vi "Morse_Decoder.vi"() -> ()   [LabVIEW 2024]
uses:
  <vilib>/DAQmx/read.llb/DAQmx Read (Analog 2D DBL NChan NSamp).vi
  <vilib>/DAQmx/create/channels.llb/DAQmx Create Channel (AI-Voltage-Basic).vi
  <vilib>/DAQmx/configure/timing.llb/DAQmx Timing (Sample Clock).vi
  <vilib>/DAQmx/miscellaneous.llb/DAQmx Fill In Error Info.vi
panel:
  out "output variable":i32[](array[numeric])
  out "String Pre Procesare":string
  out "result_out":i32[](array[numeric])
  out "size(s)":i32
  out "result_len":i32
  out "morse_len":dbl
  in  "Tab Control":enum32{"TAB"}(tab)
  out "Decoded message":i16[](graph)
  out "Trigger view":waveform(dbl)(graph)={"t0"=timestamp(0 s since 1904-01-01), "dt"=0.0002, "Y"=[]}
  out "TX":bool
  in  "StartRX":bool=TRUE
  in  "ClearMsgBuffer":bool
  in  "STOP":bool
  in  "sample mode":i32(ring)=10178 items=["Finite Samples"=10178, "Continuous Samples"=10123, "Hardware Timed Single Point"=12522]
  in  "physical channels":tag="Dev2/ai0"
  in  "input terminal configuration":i32(ring)=10083 items=["default"=-1, "RSE"=10083, "NRSE"=10078, "Differential"=10106, "Pseudodifferential"=12529]
  in  "maximum value":dbl=5.0 format="%0.2f"
  in  "minimum value":dbl=-5.0 format="%0.2f"
  in  "milliseconds to wait":u32=10
  in  "Prag":dbl(knob)=0.1 scale=0.0..5.0
  in  "samples per channel":i32=50
  in  "rate":dbl=5000.0 format="%0.2f"
  in  "timeout":dbl=10.0 format="%0.2f"
  in  "number of samples per channel":i32=50
  out "perioada":dbl
  out "error out":errorcluster
  out "MESSAGE ARRAY SIZE":i32
  out "READ BUFFER SIZE":i32=302
  out "TXStopBuff":dbl=24.0
  out "INTERMIDIATE BUFFER":dbl[](array[numeric])
  out "READ BUFFER":dbl[](array[numeric])
  out "MESSAGE ARRAY":bool[](array[boolean])
  out "Message points":bool[](array[boolean])
  out "dbg lamp":bool
  out "TrueCnt":i32
  in  "Clear String":bool
  out "Message":string
  # "INPUT CONFIG"
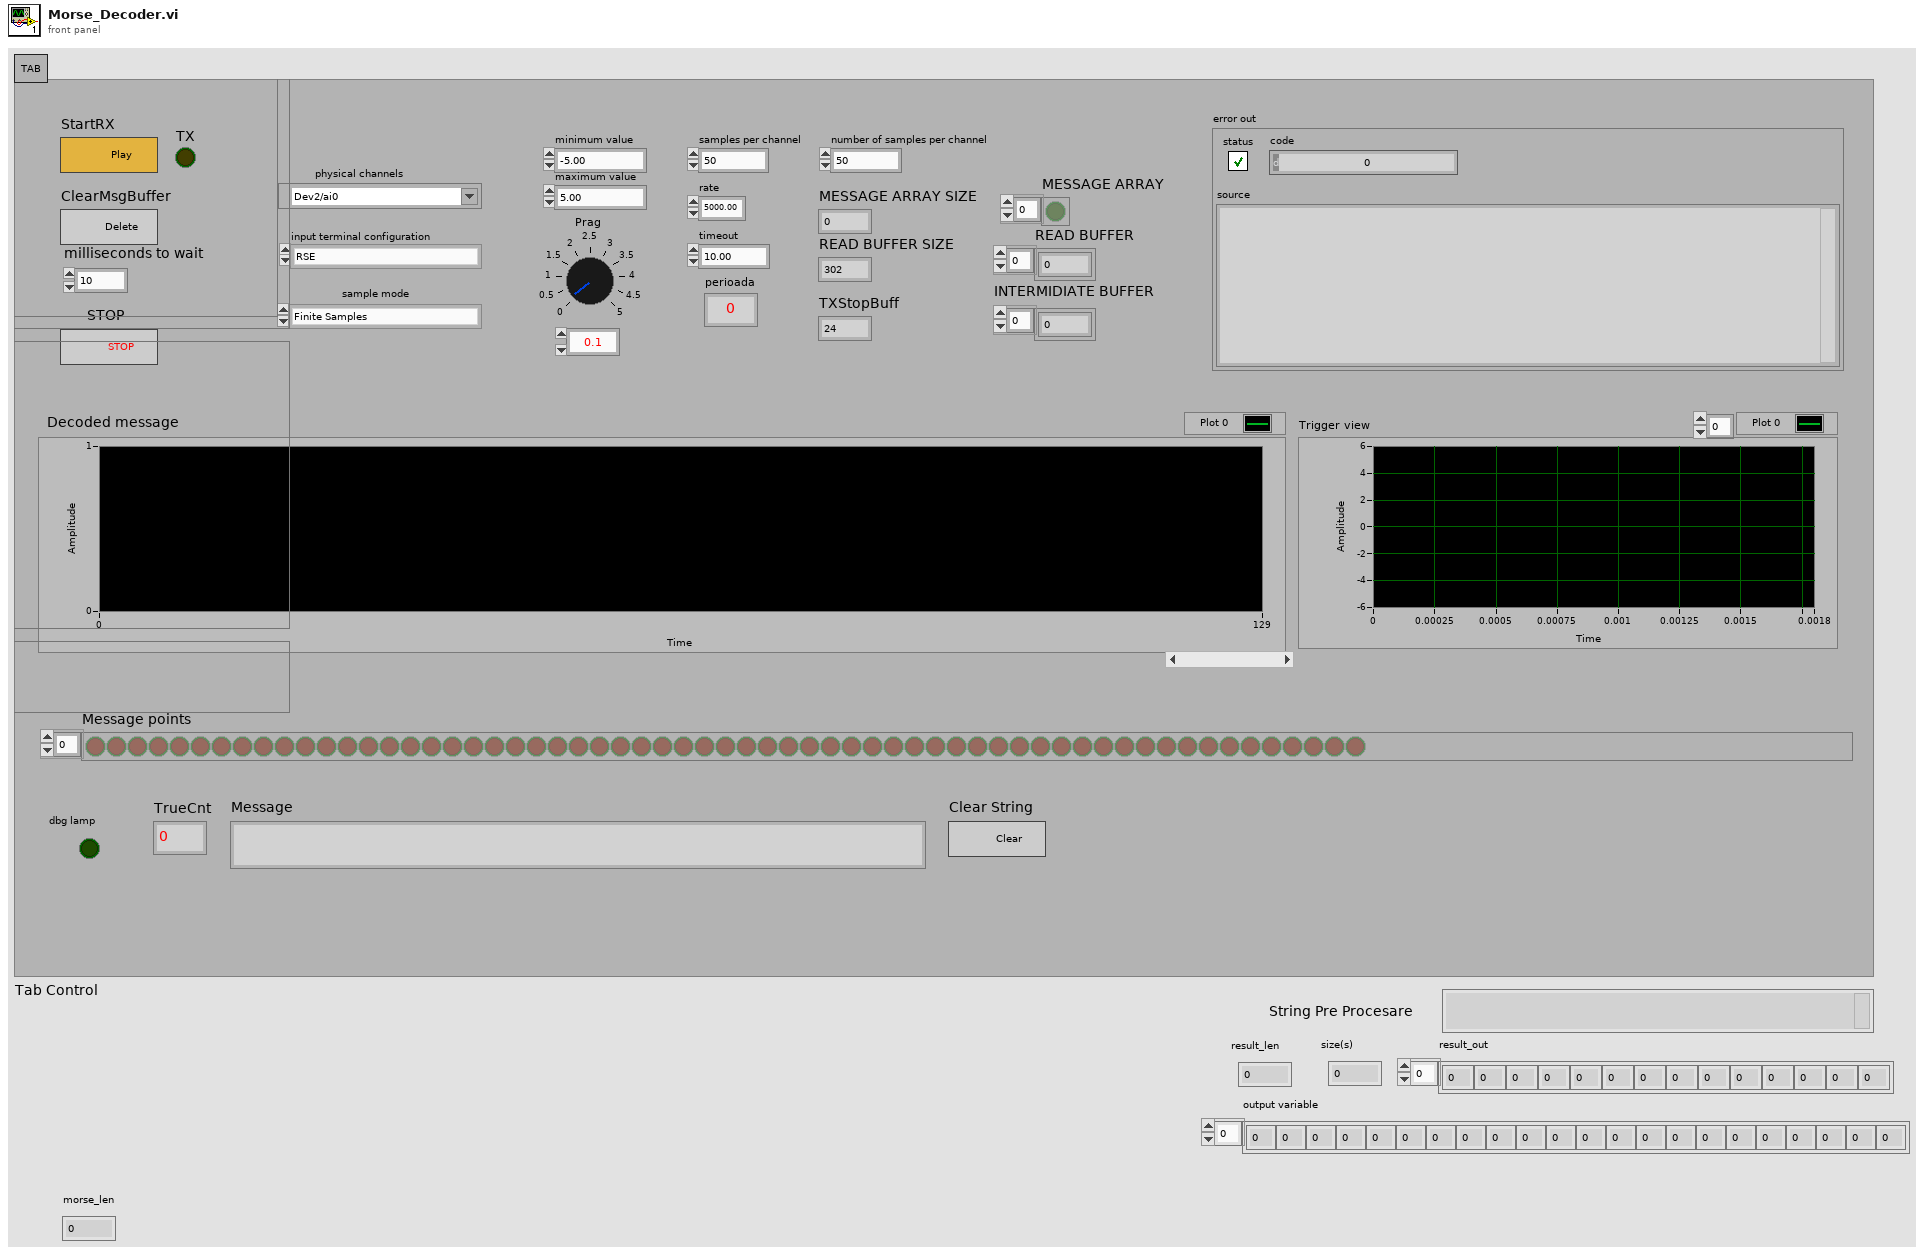
[diagram p1: front panel]
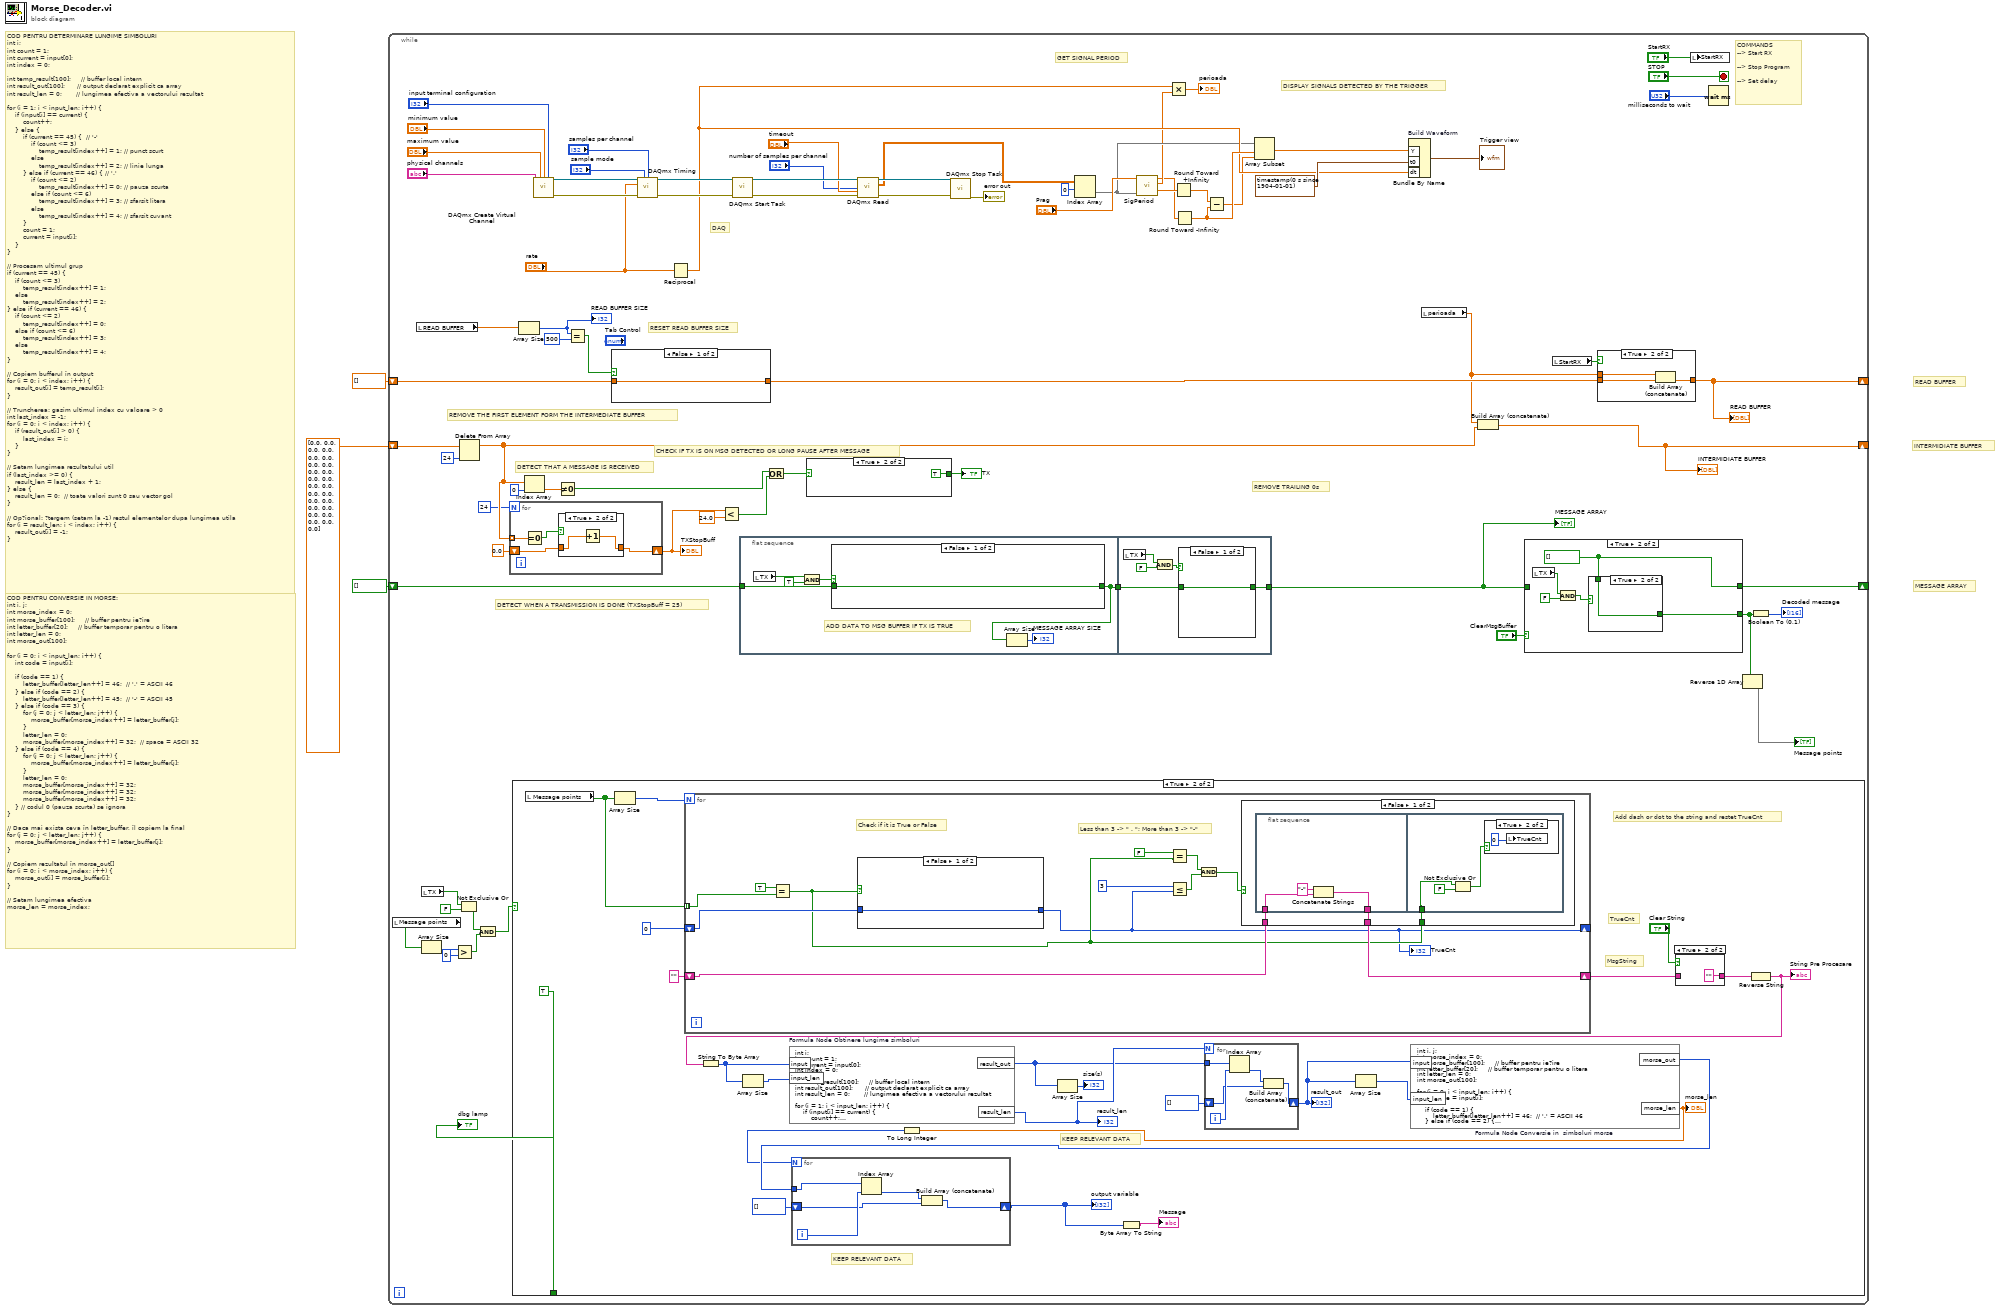
[diagram p0: block diagram]
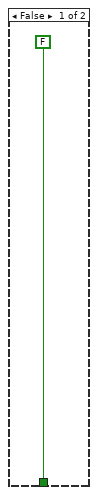
[diagram p2: hidden frame]
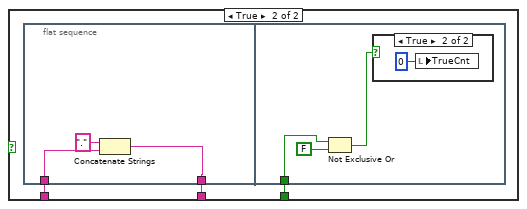
[diagram p5: hidden frame]
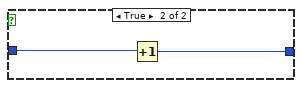
[diagram p7: hidden frame]
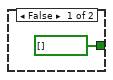
[diagram p9: hidden frame]
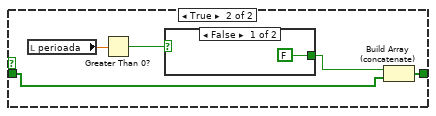
[diagram p10: hidden frame]
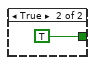
[diagram p11: hidden frame]
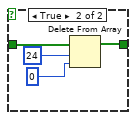
[diagram p12: hidden frame]
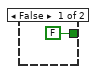
[diagram p15: hidden frame]
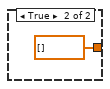
[diagram p16: hidden frame]
diagram:
  # "COD PENTRU CONVERSIE IN MORSE:\nint i, j;\nint morse_index = 0;\nint morse_buffer[100];     // buffer pentru ie?ire\nint letter_buffer[20];     // buffer temporar pentru o litera\nint letter_len = 0;\nint morse_out[100];\n\nfor (i = 0; i < input_len; i++) {\n    int code = input[i];\n\n    if (code == 1) {\n        letter_buffer[letter_len++] = 46;  // '.' = ASCII 46\n    } else if (code == 2) {\n        letter_buffer[letter_len++] = 45;  // '-' = ASCII 45\n    } else if (code == 3) {\n        for (j = 0; j < letter_len; j++) {\n            morse_buffer[morse_index++] = letter_buffer[j];\n        }\n        letter_len = 0;\n        morse_buffer[morse_index++] = 32;  // space = ASCII 32\n    } else if (code == 4) {\n        for (j = 0; j < letter_len; j++) {\n            morse_buffer[morse_index++] = letter_buffer[j];\n        }\n        letter_len = 0;\n        morse_buffer[morse_index++] = 32;\n        morse_buffer[morse_index++] = 32;\n        morse_buffer[morse_index++] = 32;\n    } // codul 0 (pauza scurta) se ignora\n}\n\n// Daca mai exista ceva în letter_buffer, îl copiem la final\nfor (j = 0; j < letter_len; j++) {\n    morse_buffer[morse_index++] = letter_buffer[j];\n}\n\n// Copiem rezultatul în morse_out[]\nfor (i = 0; i < morse_index; i++) {\n    morse_out[i] = morse_buffer[i];\n}\n\n// Setam lungimea efectiva\nmorse_len = morse_index;"
  # "COD PENTRU DETERMINARE LUNGIME SIMBOLURI\nint i;\nint count = 1;\nint current = input[0];\nint index = 0;\n\nint temp_result[100];     // buffer local intern\nint result_out[100];      // output declarat explicit ca array\nint result_len = 0;       // lungimea efectiva a vectorului rezultat\n\nfor (i = 1; i < input_len; i++) {\n    if (input[i] == current) {\n        count++;\n    } else {\n        if (current == 45) {  // '-'\n            if (count <= 3)\n                temp_result[index++] = 1; // punct scurt\n            else\n                temp_result[index++] = 2; // linie lunga\n        } else if (current == 46) { // '.'\n            if (count <= 2)\n                temp_result[index++] = 0; // pauza scurta\n            else if (count <= 6)\n                temp_result[index++] = 3; // sfarsit litera\n            else\n                temp_result[index++] = 4; // sfarsit cuvant\n        }\n        count = 1;\n        current = input[i];\n    }\n}\n\n// Procesam ultimul grup\nif (current == 45) {\n    if (count <= 3)\n        temp_result[index++] = 1;\n    else\n        temp_result[index++] = 2;\n} else if (current == 46) {\n    if (count <= 2)\n        temp_result[index++] = 0;\n    else if (count <= 6)\n        temp_result[index++] = 3;\n    else\n        temp_result[index++] = 4;\n}\n\n// Copiem bufferul în output\nfor (i = 0; i < index; i++) {\n    result_out[i] = temp_result[i];\n}\n\n// Truncherea: gasim ultimul index cu valoare > 0\nint last_index = -1;\nfor (i = 0; i < index; i++) {\n    if (result_out[i] > 0) {\n        last_index = i;\n    }\n}\n\n// Setam lungimea rezultatului util\nif (last_index >= 0) {\n    result_len = last_index + 1;\n} else {\n    result_len = 0;  // toate valori sunt 0 sau vector gol\n}\n\n// Op?ional: ?tergem (setam la -1) restul elementelor dupa lungimea utila\nfor (i = result_len; i < index; i++) {\n    result_out[i] = -1;\n}"
  # "INTERMIDIATE BUFFER"
  # "READ BUFFER"
  # "MESSAGE ARRAY"
  n1 = while {
    shift-right: [w17] -> _
    shift-left: bool[] [] -> [w20]
    shift-right: [w44] -> _
    shift-left: dbl[] [] -> [w41]
    shift-right: [w35] -> _
    shift-left: dbl[] [0.0, 0.0, 0.0, 0.0, 0.0, 0.0, 0.0, 0.0, 0.0, 0.0, 0.0, 0.0, 0.0, 0.0, 0.0, 0.0, 0.0, 0.0, 0.0, 0.0, 0.0, 0.0, 0.0, 0.0, 0.0] -> [w36]
    stop <- "STOP" stop-if-true
    # "REMOVE TRAILING 0s"
    # "COMMANDS\n--> Start RX\n\n--> Stop Program\n\n--> Set delay"
    # "REMOVE THE FIRST ELEMENT FORM THE INTERMEDIATE BUFFER"
    # "DAQ"
    # "GET SIGNAL PERIOD"
    # "DISPLAY SIGNALS DETECTED BY THE TRIGGER"
    # "CHECK IF TX IS ON MSG DETECTED OR LONG PAUSE AFTER MESSAGE"
    # "DETECT WHEN A TRANSMISSION IS DONE (TXStopBuff = 25)"
    # "DETECT THAT A MESSAGE IS RECEIVED"
    # "RESET READ BUFFER SIZE"
    n2 = local read "Message points"() -> (w10:bool[])
    n3 = local read "READ BUFFER"() -> (w39:dbl[])
    n4 = local read "TX"() -> (w11:bool)
    n5 = Array Size(array=w10) -> (size(s)=w9:i32)
    n6 = Greater?(x=w9, y=0) -> (0:w6:bool)
    n7 = Not Exclusive Or(1:FALSE ("y"), 2:w11) -> (0:w7:bool)
    n8 = Delete From Array(array=w36, index=24) -> (array with subset deleted=w30:dbl[])  [unwired: 1 in, 1 out]
    n9 = And(x=w7, y=w6) -> (x .and. y?=w5:bool)
    n10 = for {
      N: 24 -> [_]
      shift-right: [w187] -> w25
      shift-left: 0.0 -> [w188]
      tunnel: w30 -> [w190] mode=indexing
      n11 = Equal To 0?(x=w190) -> (x = 0?=w189:bool)
      n12 = case shown="True" w189 {
        tunnel: w188 -> [w191 w193]
        tunnel: [w191 w192] -> w187
        frame False {
        }
        frame True {
          n13 = Increment(x=w193) -> (x+1=w192:dbl)
        }
      }
    }
    "TXStopBuff" <- w25
    n14 = case shown="True" w5 {
      tunnel: [FALSE TRUE] -> w4
      frame False {
      }
      frame True {
        # "KEEP RELEVANT DATA"
        # "KEEP RELEVANT DATA"
        # "Add dash or dot to the string and restet TrueCnt"
        # "MsgString"
        # "TrueCnt"
        n15 = local read "Message points"() -> (w101:bool[])
        n16 = Array Size(array=w101) -> (size(s)=w103:i32)
        n17 = for {
          N: w103 -> [_]
          shift-right: [w122] -> w100
          shift-left: "" -> [w123]
          shift-right: [w116] -> _
          shift-left: 0 -> [w125]
          tunnel: w101 -> [w127] mode=indexing
          # "Less than 3 -> \" . \"; More than 3 -> \"-\""
          # "Check if it is True or False"
          n18 = Equal?(x=TRUE, y=w127) -> (x = y?=w121:bool)
          n19 = case shown="False" w121 {
            tunnel: w125 -> [w148 w150]
            tunnel: [w148 w149] -> w116
            frame False {
            }
            frame True {
              n20 = Increment(x=w150) -> (x+1=w149:i32)
            }
          }
          "TrueCnt" <- w116
          n21 = Equal?(x=FALSE, y=w121) -> (x = y?=w119:bool)
          n22 = Less Or Equal?(x=3, y=w116) -> (x <= y?=w118:bool)
          n23 = And(x=w119, y=w118) -> (x .and. y?=w117:bool)
          n24 = case shown="False" w117 {
            tunnel: w123 -> [w130 w140]
            tunnel: [w129 w139] -> w122
            tunnel: w121 -> [w128 w138]
            frame False {
              n25 = flat-sequence {
                tunnel: w130 -> [w133]
                tunnel: [w132] -> w129
                tunnel: w128 -> [w134]
                frame #0 {
                  n26 = Concatenate Strings("-" ("string"), w133) -> (w132:string)
                }
                frame #1 {
                  n27 = Not Exclusive Or(1:FALSE ("y"), 2:w134) -> (0:w136:bool)
                  n28 = case shown="True" w136 {
                    frame False {
                    }
                    frame True {
                      n29 = local write "TrueCnt"(0) -> ()
                    }
                  }
                }
              }
            }
            frame True {
              n30 = flat-sequence {
                tunnel: [w142] -> w139
                tunnel: w140 -> [w143]
                tunnel: w138 -> [w144]
                frame #0 {
                  n31 = Concatenate Strings("." ("string"), w143) -> (w142:string)
                }
                frame #1 {
                  n32 = Not Exclusive Or(1:FALSE ("y"), 2:w144) -> (0:w146:bool)
                  n33 = case shown="True" w146 {
                    frame False {
                    }
                    frame True {
                      n34 = local write "TrueCnt"(0 ("TrueCnt")) -> ()
                    }
                  }
                }
              }
            }
          }
        }
        n35 = case shown="True" "Clear String" {
          tunnel: w100 -> [w114 _]
          tunnel: [w114 ""] -> w97
          frame False {
          }
          frame True {
          }
        }
        n36 = Reverse String(1:w97) -> (0:w93:string)
        "String Pre Procesare" <- w93
        n37 = String To Byte Array(string=w93) -> (unsigned byte array=w95:u8[])
        n38 = Array Size(array=w95) -> (size(s)=w94:i32)
        n39 = formula code="int i;\nint count = 1;\nint current = input[0];\nint index = 0;\n\nint temp_result[100];     // buffer local intern\nint result_out[100];      // output declarat explicit ca array\nint result_len = 0;       // lungimea efectiva a vectorului rezultat\n\nfor (i = 1; i < input_len; i++) {\n    if (input[i] == current) {\n        count++;\n    } else {\n        if (current == 45) {  // '-'\n            if (count <= 3)\n                temp_result[index++] = 1; // punct scurt\n            else\n                temp_result[index++] = 2; // linie lunga\n        } else if (current == 46) { // '.'\n            if (count <= 2)\n                temp_result[index++] = 0; // pauza scurta\n            else if (count <= 6)\n                temp_result[index++] = 3; // sfarsit litera\n            else\n                temp_result[index++] = 4; // sfarsit cuvant\n        }\n        count = 1;\n        current = input[i];\n    }\n}\n\n// Procesam ultimul grup\nif (current == 45) {\n    if (count <= 3)\n        temp_result[index++] = 1;\n    else\n        temp_result[index++] = 2;\n} else if (current == 46) {\n    if (count <= 2)\n        temp_result[index++] = 0;\n    else if (count <= 6)\n        temp_result[index++] = 3;\n    else\n        temp_result[index++] = 4;\n}\n\n// Copiem bufferul în output\nfor (i = 0; i < index; i++) {\n    result_out[i] = temp_result[i];\n}\n\n// Truncherea: gasim ultimul index cu valoare > 0\nint last_index = -1;\nfor (i = 0; i < index; i++) {\n    if (result_out[i] > 0) {\n        last_index = i;\n    }\n}\n\n// Setam lungimea rezultatului util\nif (last_index >= 0) {\n    result_len = last_index + 1;\n} else {\n    result_len = 0;  // toate valori sunt 0 sau vector gol\n}\n\n// Op?ional: ?tergem (setam la -1) restul elementelor dupa lungimea utila\nfor (i = result_len; i < index; i++) {\n    result_out[i] = -1;\n}" "Formula Node Obtinere lungime simboluri"("input"=w95, "input_len"=w94) -> ("result_out"=w90:i32[], "result_len"=w91:i32)
        "result_len" <- w91
        n40 = Array Size(array=w90) -> (size(s)=→"size(s)":i32)
        n41 = for {
          N: w91 -> [_]
          tunnel: w90 -> [w112]
          shift-right: [w109] -> w88
          shift-left: i32[] [] -> [w110]
          i -> [w113]
          n42 = Index Array(array=w112, index=w113) -> (element=w111:i32)
          n43 = Build Array (concatenate)(w111, w110) -> (w109:i32[])
        }
        "result_out" <- w88
        n44 = Array Size(array=w88) -> (size(s)=w87:i32)
        n45 = formula code="int i, j;\nint morse_index = 0;\nint morse_buffer[100];     // buffer pentru ie?ire\nint letter_buffer[20];     // buffer temporar pentru o litera\nint letter_len = 0;\nint morse_out[100];\n\nfor (i = 0; i < input_len; i++) {\n    int code = input[i];\n\n    if (code == 1) {\n        letter_buffer[letter_len++] = 46;  // '.' = ASCII 46\n    } else if (code == 2) {\n        letter_buffer[letter_len++] = 45;  // '-' = ASCII 45\n    } else if (code == 3) {\n        for (j = 0; j < letter_len; j++) {\n            morse_buffer[morse_index++] = letter_buffer[j];\n        }\n        letter_len = 0;\n        morse_buffer[morse_index++] = 32;  // space = ASCII 32\n    } else if (code == 4) {\n        for (j = 0; j < letter_len; j++) {\n            morse_buffer[morse_index++] = letter_buffer[j];\n        }\n        letter_len = 0;\n        morse_buffer[morse_index++] = 32;\n        morse_buffer[morse_index++] = 32;\n        morse_buffer[morse_index++] = 32;\n    } // codul 0 (pauza scurta) se ignora\n}\n\n// Daca mai exista ceva în letter_buffer, îl copiem la final\nfor (j = 0; j < letter_len; j++) {\n    morse_buffer[morse_index++] = letter_buffer[j];\n}\n\n// Copiem rezultatul în morse_out[]\nfor (i = 0; i < morse_index; i++) {\n    morse_out[i] = morse_buffer[i];\n}\n\n// Setam lungimea efectiva\nmorse_len = morse_index;" "Formula Node Conversie in  simboluri morse"("input"=w88, "input_len"=w87) -> ("morse_out"=w85:i32[], "morse_len"=w84:dbl)
        "morse_len" <- w84
        n46 = To Long Integer(number=w84) -> (32bit integer=w83:i32)
        n47 = for {
          N: w83 -> [_]
          shift-right: [w106] -> w81
          shift-left: i32[] [] -> [w104]
          tunnel: w85 -> [w108]
          i -> [w107]
          n48 = Index Array(array=w108, index=w107) -> (element=w105:i32)
          n49 = Build Array (concatenate)(w105, w104) -> (w106:i32[])
        }
        "output variable" <- w81
        n50 = Byte Array To String(unsigned byte array=w81) -> (string=→"Message":string)
      }
    }
    "dbg lamp" <- w4
    n51 = Array Size(array=w39) -> (size(s)=w38:i32)
    "READ BUFFER SIZE" <- w38
    n52 = Index Array(array=w30, index=0) -> (element=w33:dbl)
    n53 = call-poly <vilib>:"DAQmx Create Virtual Channel.vi"("maximum value"="maximum value", "minimum value"="minimum value", "input terminal configuration"="input terminal configuration", "physical channels"="physical channels") -> ("task out"=w74:refnum<k21>, "error out"=w79:errorcluster)  [unwired: 10 in]
    n54 = Not Equal To 0?(x=w33) -> (x != 0?=w26:bool)
    n55 = Equal?(x=w38, y=500) -> (x = y?=w42:bool)
    n56 = case shown="False" w42 {
      tunnel: w41 -> [w196 _]
      tunnel: [w196 dbl[] []] -> w40
      frame False {
      }
      frame True {
      }
    }
    n57 = call-poly <vilib>:"DAQmx Timing.vi"("task/channels in"=w74, "sample mode"="sample mode", "samples per channel"="samples per channel", "rate"="rate", "error in"=w79) -> ("task out"=w73:refnum<k21>, "error out"=w78:errorcluster)  [unwired: 9 in]
    n58 = Reciprocal(x="rate") -> (1/x=w54:dbl)
    n59 = Less?(x=w25, y=24.0) -> (x < y?=w23:bool)
    n60 = call <vilib>:"DAQmx Start Task.vi"("task/channels in"=w73, "error in"=w78) -> ("task out"=w72:refnum<k21>, "error out"=w77:errorcluster)  [unwired: 12 in]
    n61 = flat-sequence {
      tunnel: w20 -> [w163]
      tunnel: [w159] -> w19
      tunnel: w19 -> [w174]
      tunnel: [w173] -> w15
      frame #0 {
        # "ADD DATA TO MSG BUFFER IF TX IS TRUE"
        n62 = local read "TX"() -> (w160:bool)
        n63 = And(x=w160, y=TRUE) -> (x .and. y?=w162:bool)
        n64 = case shown="False" w162 {
          tunnel: [w165 w170] -> w159
          tunnel: w163 -> [w165 w166]
          frame False {
          }
          frame True {
            n65 = local read "perioada"() -> (w168:dbl)
            n66 = Greater Than 0?(x=w168) -> (x > 0?=w169:bool)
            n67 = case shown="False" w169 {
              tunnel: [FALSE TRUE] -> w167
              frame False {
              }
              frame True {
              }
            }
            n68 = Build Array (concatenate)(w167, w166) -> (w170:bool[])
          }
        }
        n69 = Array Size(array=w159) -> (size(s)=→"MESSAGE ARRAY SIZE":i32)
      }
      frame #1 {
        n70 = local read "TX"() -> (w177:bool)
        n71 = And(x=w177, y=FALSE) -> (x .and. y?=w175:bool)
        n72 = case shown="False" w175 {
          tunnel: w174 -> [w178 w182]
          tunnel: [w178 w179] -> w173
          frame False {
          }
          frame True {
            n73 = Delete From Array(array=w182, length=24, index=0) -> (array with subset deleted=w179:bool[])  [unwired: 1 out]
          }
        }
      }
    }
    n74 = Or(x=w26, y=w23) -> (x .or. y?=w27:bool)
    n75 = case shown="True" w27 {
      tunnel: [FALSE TRUE] -> w32
      frame False {
      }
      frame True {
      }
    }
    "TX" <- w32
    n76 = call-poly <vilib>:"DAQmx Read.vi"("task/channels in"=w72, "number of samples per channel"="number of samples per channel", "timeout"="timeout", "error in"=w77) -> ("task out"=w71:refnum<k21>, "data"=w60:dbl[][], "error out"=w76:errorcluster)  [unwired: 9 in]
    n77 = call <vilib>:"DAQmx Stop Task.vi"("task/channels in"=w71, "error in"=w76) -> ("error out"=→"error out":errorcluster)  [unwired: 12 in, 1 out]
    n78 = Index Array "Index Array"(array=w60, index (row)=0 ("index")) -> (element=w51:dbl[])  [unwired: 1 in]
    n79 = call "SigPeriod.vi"("Array"=w51, "Prag"="Prag") -> ("Ultimul Punct"=w48:dbl, "Perioada"=w49:dbl, "Primul PUNCT"=w47:dbl)  [unwired: 7 in]
    n80 = Multiply(x=w54, y=w49) -> (x*y=→"perioada":dbl)
    n81 = Round Toward +Infinity(x=w48) -> (ceil(x): smallest int >= x=w58:dbl)
    n82 = Round Toward -Infinity(1:w47) -> (0:w56:dbl)
    n83 = Subtract(x=w58, y=w56) -> (x-y=w53:dbl)
    n84 = Array Subset "Array Subset"(array=w51, index=w56, length=w53) -> (w52:dbl[])
    n85 = Bundle By Name "Build Waveform"("Y"=w52, "t0"=timestamp(0 s since 1904-01-01), "dt"=w54) -> (→"Trigger view":waveform(dbl))  [unwired: 1 in]
    n86 = local read "perioada"() -> (w37:dbl)
    n87 = Build Array (concatenate)(w37, w30) -> (w35:dbl[])
    "INTERMIDIATE BUFFER" <- w35
    n88 = case shown="True" "ClearMsgBuffer" {
      tunnel: w15 -> [w151 _]
      tunnel: [w151 w153] -> w17
      tunnel: [w151 w152] -> w14
      frame False {
      }
      frame True {
        w153 = bool[] []
        n89 = local read "TX"() -> (w155:bool)
        n90 = And(x=w155, y=FALSE) -> (x .and. y?=w154:bool)
        n91 = case shown="True" w154 {
          tunnel: w153 -> [_ w158]
          tunnel: [bool[] [] w158] -> w152
          frame False {
          }
          frame True {
          }
        }
      }
    }
    n92 = local read "StartRX"() -> (w21:bool)
    n93 = case shown="True" w21 {
      tunnel: [w183 w186] -> w44
      tunnel: w40 -> [w183 w185]
      tunnel: w37 -> [_ w184]
      frame False {
      }
      frame True {
        n94 = Build Array (concatenate)(w184, w185) -> (w186:dbl[])
      }
    }
    "READ BUFFER" <- w44
    n95 = local write "StartRX"("StartRX") -> ()
    n96 = Wait (ms)(milliseconds to wait="milliseconds to wait") -> ()  [unwired: 1 out]
    n97 = Reverse 1D Array(array=w14) -> (reversed array=→"Message points":bool[])
    n98 = Boolean To (0,1)(Boolean=w14) -> (0, 1=→"Decoded message":i16[])
    "MESSAGE ARRAY" <- w15
  }
